vi "sv_Design Octave Filter Set.vi"(0 "scaled signal [EU]":waveform(dbl), 5 "1/n octave settings":T2, 7 "band number":cluster{"low band":i32, "high band":i32}, 11 "error in (no error)":errorcluster) -> (4 "dup scaled signal [EU]":waveform(dbl), 6 "filter bank parameters":T3 {"standard filter bandwidth" format="%.2f"; "special filter bandwidth" format="%.2f"; "lowpass filter coefficients"."Forward Coefficients" format="%.2f"; "lowpass filter coefficients"."Reverse Coefficients" format="%.2f"; "standard filter coefficients"."Forward Coefficients" format="%.2f"; "standard filter coefficients"."Reverse Coefficients" format="%.2f"; "special filter coefficients"."Forward Coefficients" format="%.2f"; "special filter coefficients"."Reverse Coefficients" format="%.2f"}, 8 "initial filter state":T4 {"result" format="%.2f"; "linear averaging"."size" format="%.2f"; "linear averaging"."squared sum" format="%.2f"; "exponential averaging"."peak detector" format="%.2f"; "exponential averaging"."exponential averaging" format="%.2f"; "lowpass filter" format="%.2f"; "octave filter"."Octave filter" format="%.2f"}, 10 "nominal frequencies [Hz]":dbl[](array[numeric]) format="%.2f", 15 "error out":errorcluster)   [LabVIEW 2017, in "SoundVib_Octave.lvlib"]
uses:
  <vilib>/addons/Sound and Vibration/svt_Octave/SoundVib_Octave.lvlib
  <vilib>/addons/_NISVFA/_Shared subVIs/Controls/svc_Octave Standard.ctl
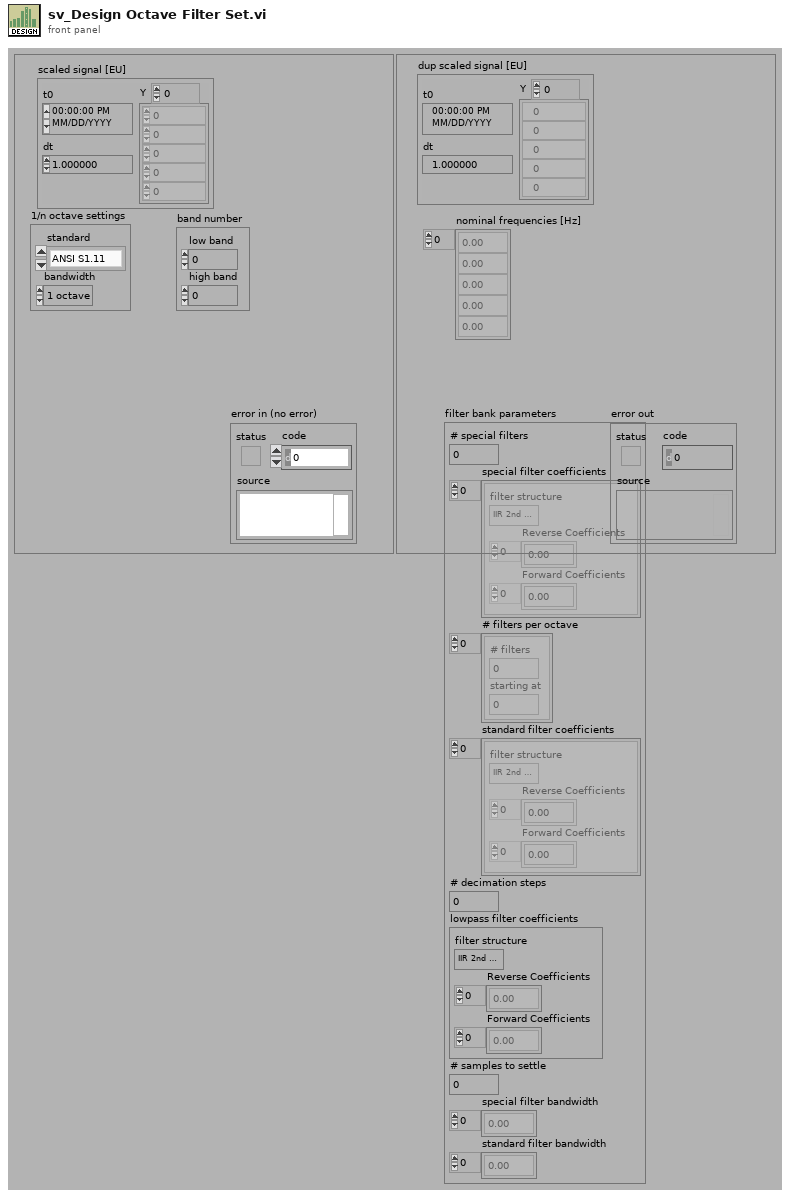
[diagram p1: front panel]
types:
  T1 = typedef "svc_Octave Standard.ctl" = enum16{"ANSI S1.11", "IEC 61260"}
  T2 = cluster{"standard":T1, "bandwidth":enum16{"1 octave", "1/3 octave", "1/6 octave", "1/12 octave", "1/24 octave"}}
  T3 = cluster{"# special filters":i32, "special filter coefficients":cluster{"filter structure":enum32{"IIR 2nd Order", "IIR 4th Order"}, "Reverse Coefficients":dbl[], "Forward Coefficients":dbl[]}[], "# filters per octave":cluster{"# filters":i32, "starting at":i32}[], "standard filter coefficients":cluster{"filter structure":enum32{"IIR 2nd Order", "IIR 4th Order"}, "Reverse Coefficients":dbl[], "Forward Coefficients":dbl[]}[], "# decimation steps":i32, "lowpass filter coefficients":cluster{"filter structure":enum32{"IIR 2nd Order", "IIR 4th Order"}, "Reverse Coefficients":dbl[], "Forward Coefficients":dbl[]}, "# samples to settle":u64, "special filter bandwidth":dbl[], "standard filter bandwidth":dbl[]}
  T4 = cluster{"octave filter":cluster{"Octave filter":dbl[]}[], "decimation":i32[], "lowpass filter":dbl[][], "exponential averaging":cluster{"exponential averaging":dbl, "peak detector":dbl}[], "linear averaging":cluster{"squared sum":dbl, "size":dbl}[], "result":dbl[], "# samples since init":u64}
  T5 = enum16{"1 octave", "1/3 octave", "1/6 octave", "1/12 octave", "1/24 octave"}
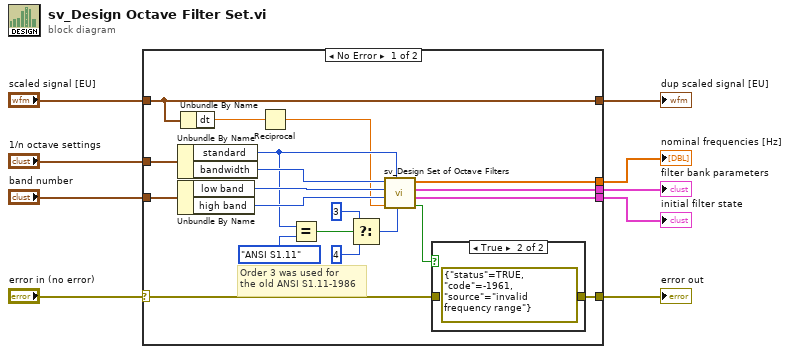
[diagram p0: block diagram]
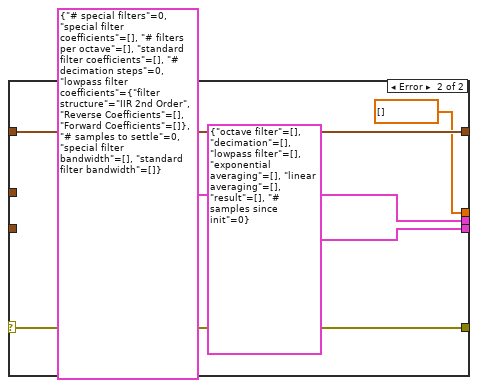
[diagram p3: hidden frame]
diagram:
  n1 = case shown="No Error" "error in (no error)" {
    selector: "error in (no error)" -> [w13 w32]
    tunnel: [w29 dbl[] [] ("nominal frequencies [Hz]")] -> w9
    tunnel: [w28 T4 {"octave filter"=[], "decimation"=[], "lowpass filter"=[], "exponential averaging"=[], "linear averaging"=[], "result"=[], "# samples since init"=0} ("initialize filter state")] -> w8
    tunnel: [w27 T3 {"# special filters"=0, "special filter coefficients"=[], "# filters per octave"=[], "standard filter coefficients"=[], "# decimation steps"=0, "lowpass filter coefficients"={"filter structure"=enum."IIR 2nd Order", "Reverse Coefficients"=[], "Forward Coefficients"=[]}, "# samples to settle"=0, "special filter bandwidth"=[], "standard filter bandwidth"=[]} ("filter bank parameters")] -> w7
    tunnel: "band number" -> [w26 _]
    tunnel: "1/n octave settings" -> [w25 _]
    tunnel: "scaled signal [EU]" -> [w15 w36]
    tunnel: [w14 w32] -> w2
    tunnel: [w15 w36] -> w1
    frame No Error {
      # "Order 3 was used for\nthe old ANSI S1.11-1986"
      n2 = Unbundle By Name(w25) -> ("standard"=w11:T1, "bandwidth"=w20:T5)
      n3 = Unbundle By Name(w26) -> ("low band"=w21:i32, "high band"=w22:i32)
      n4 = Unbundle By Name(w15) -> ("dt"=w24:dbl)
      n5 = Reciprocal(x=w24) -> (1/x=w10:dbl)
      n6 = Equal?(x=w11, y=svc_Octave_Standard."ANSI S1.11") -> (x = y?=w17:bool)
      n7 = Select(t=3 ("Butterworth filter order"), s=w17, f=4) -> (s? t:f=w23:i32)
      n8 = call <vilib>:"sv_Design Set of Octave Filters.vi"("Butterworth filter order"=w23, "standard"=w11, "sampling frequency [Hz]"=w10, "high band selector"=w22, "low band selector"=w21, "bandwidth"=w20) -> ("error"=w12:bool, "initialize filter state"=w28:T4, "filter bank parameters"=w27:T3, "nominal frequencies [Hz]"=w29:dbl[])  [unwired: 2 out]
      n9 = case shown="True" w12 {
        tunnel: w13 -> [w30 _]
        tunnel: [w30 errorcluster {"status"=TRUE, "code"=-1961, "source"="invalid frequency range"} ("error IO")] -> w14
        frame False {
        }
        frame True {
        }
      }
    }
    frame Error {
    }
  }
  "nominal frequencies [Hz]" <- w9
  "initial filter state" <- w8
  "filter bank parameters" <- w7
  "error out" <- w2
  "dup scaled signal [EU]" <- w1
